vi "Subvi sample and hold U8.vi"(8 "Clock":bool, 9 "Input":u8) -> (1 "Output":u8)   [LabVIEW 2017]
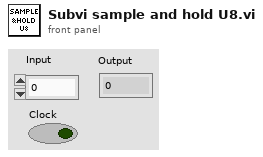
[diagram p1: front panel]
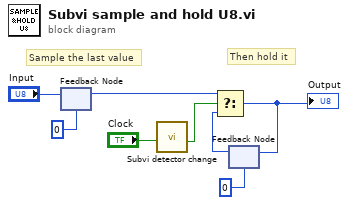
[diagram p0: block diagram]
diagram:
  # "Then hold it"
  # "Sample the last value"
  n1 = feedback #1(u8 0) -> (w5:u8)
  n2 = feedback-in #1("Input") -> ()
  n3 = call "Subvi detector change.vi"("Input"="Clock") -> ("Output"=w1:bool)  [unwired: 8 in]
  n4 = feedback #2(u8 0) -> (w4:u8)
  n5 = Select(t=w5, s=w1, f=w4) -> (s? t:f=w3:u8)
  "Output" <- w3
  n6 = feedback-in #2(w3) -> ()
